vi "Set Attribute Meta Data.vi"(6 "Meta Data":string, 7 "Unique ID":string, 8 "error in (no error)":errorcluster, 9 "Attribute Type":variant, 10 "Attribute Name":string, 11 "Test Executive Ref":refnum<data-value>) -> (0 "error out":errorcluster, 1 "Found?":bool, 3 "Test Executive Ref out":refnum<data-value>)   [LabVIEW 2017, in "Test Executive.lvlib" / "TestExecutive Ref.lvclass"]
uses:
  <vilib>/gpm_packages/@cs/test-executive/Source/Test Executive/TestExecutive Ref/TestExecutive Ref.lvclass
  <vilib>/gpm_packages/@cs/test-executive/Source/Test Executive/ITestExecutive/ITest Executive.lvclass
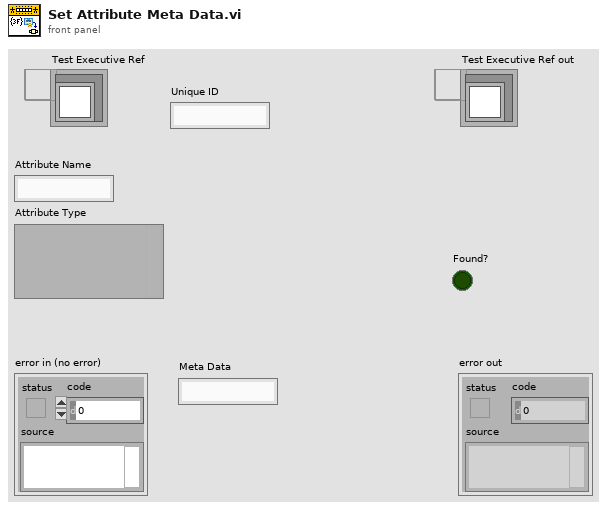
[diagram p1: front panel]
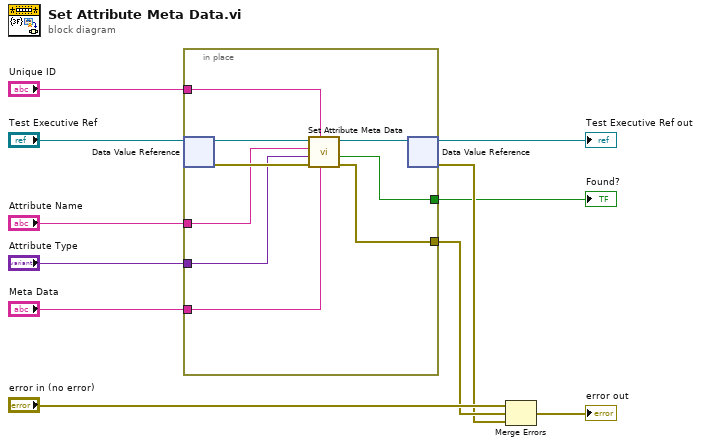
[diagram p0: block diagram]
diagram:
  n1 = in-place {
    in-place-border: "Unique ID" -> [w18]
    in-place-border: "Meta Data" -> [w12]
    in-place-border: [w16] -> w6
    in-place-border: [w15] -> w3
    in-place-border: "Attribute Name" -> [w14]
    in-place-border: "Attribute Type" -> [w13]
    n2 = in-place-dvr #1("Test Executive Ref") -> (w20:refnum<class "ITest Executive.lvclass">, w17:errorcluster)
    n3 = call-dynamic "Set Attribute Meta Data.vi"("Meta Data"=w12, "Unique ID"=w18, "error in (no error)"=w17, "Attribute Type"=w13, "Attribute Name"=w14, "ITest Executive in"=w20) -> ("error out"=w16:errorcluster, "Found?"=w15:bool, "ITest Executive out"=w19:refnum<class "ITest Executive.lvclass">)  [unwired: 3 in]
    n4 = in-place-dvr #1(w19) -> (→"Test Executive Ref out":refnum<data-value>, w5:errorcluster)
  }
  "Found?" <- w3
  n5 = Merge Errors("error in (no error)", w6, w5) -> (→"error out":errorcluster)
